vi "4.4.vi"() -> ()   [LabVIEW 2017]
panel:
  in  "数值":dbl
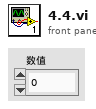
[diagram p1: front panel]
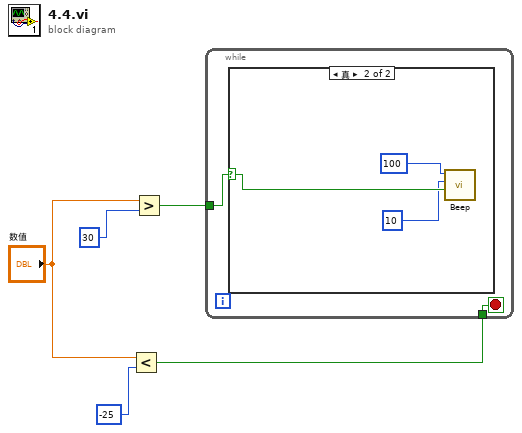
[diagram p0: block diagram]
diagram:
  n1 = Less?(x="数值", y=-25) -> (x < y?=w5:bool)
  n2 = Greater?(x="数值", y=30) -> (0:w4:bool)
  n3 = while {
    tunnel: w5 -> [w7]
    tunnel: w4 -> [w6]
    stop <- w7 stop-if-true
    n4 = case shown="真" w6 {
      selector: w6 -> [_ w10]
      frame False {
      }
      frame True {
        n5 = call <vilib>:"Beep.vi"("use system alert? (T)"=w10, "duration (msec)"=10, "frequency (Hz)"=100) -> ()  [unwired: 9 in]
      }
    }
  }
